vi "parse tcp reply and replace all device var subset.vi"(6 "All device variables array in":string[][](array[string]), 9 "regular expression":string, 10 "String":string, 11 "Clone names and reoplies in":string[][](array[string])) -> (0 "error out":errorcluster, 2 "Device Name":string, 3 "All device variables array":string[][](array[string]), 5 "Clone name and replies array":string[][](array[string]))   [LabVIEW 2020]
panel:
  out "Shot Data parsed array":string[][](array[string])
  out "tcp reply":string
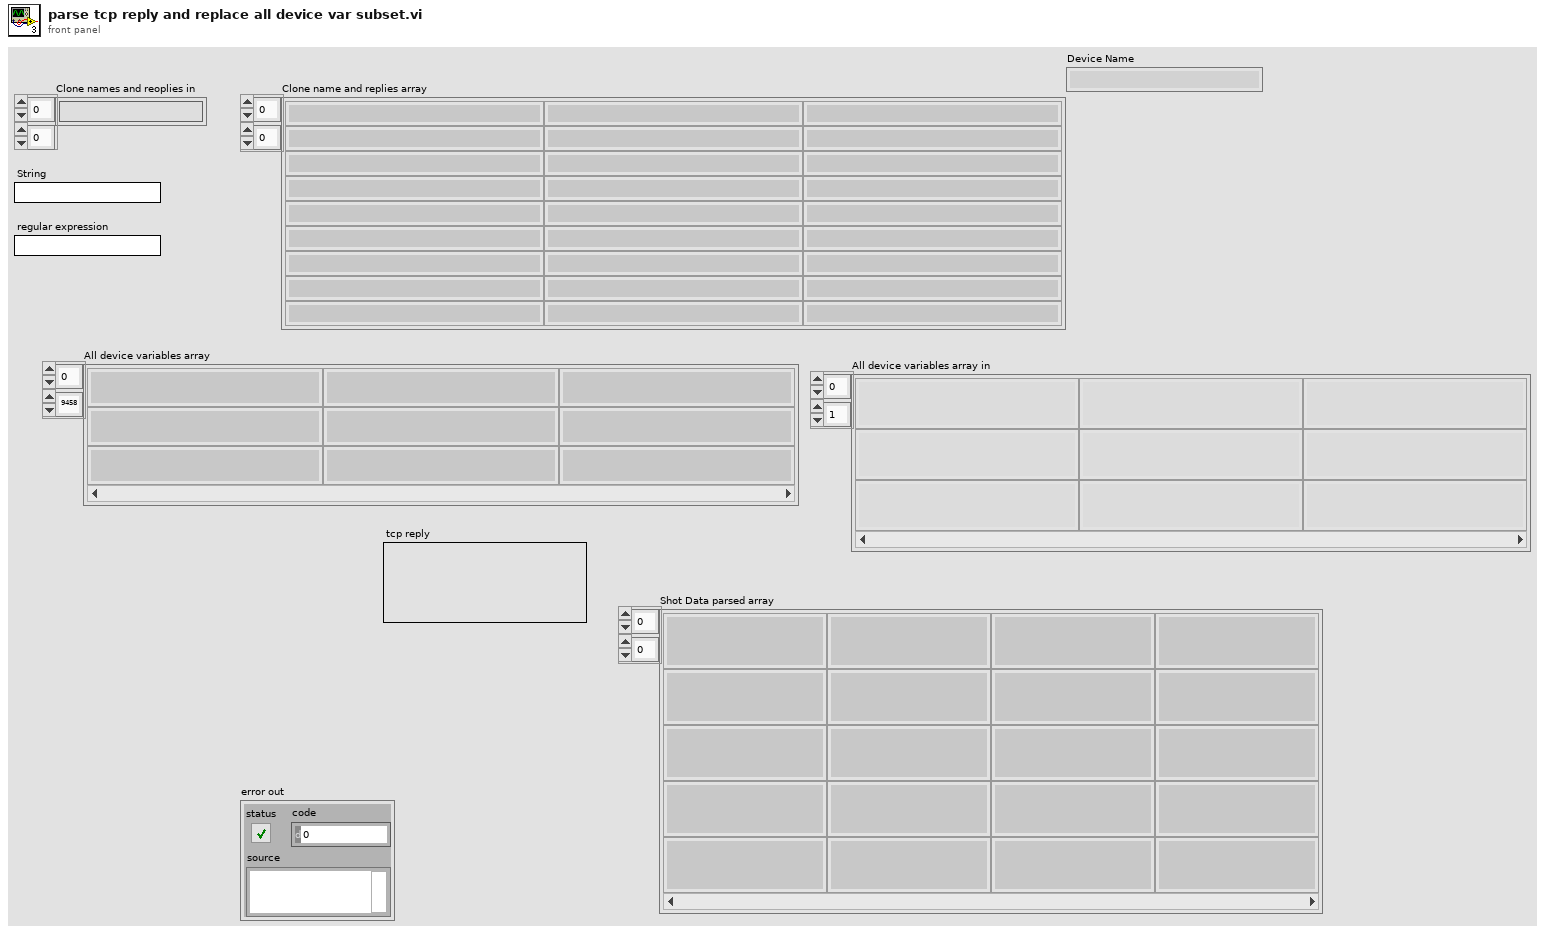
[diagram p1: front panel]
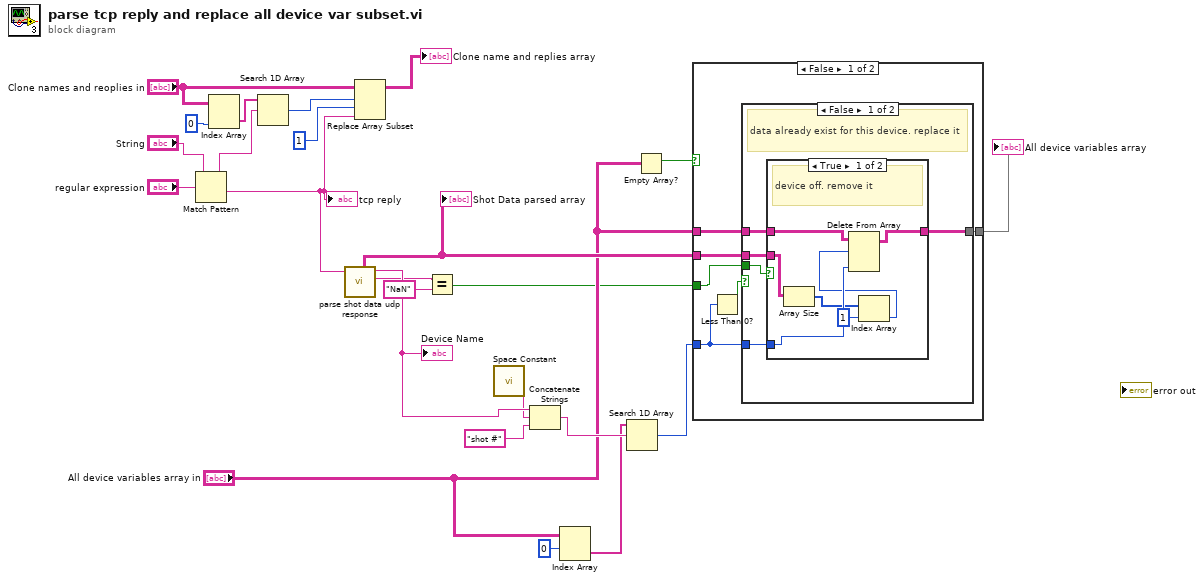
[diagram p0: block diagram]
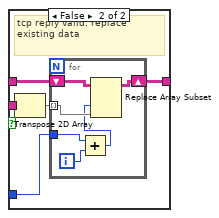
[diagram p2: hidden frame]
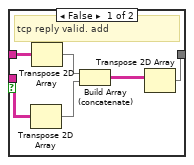
[diagram p4: hidden frame]
diagram:
  n1 = Match Pattern(string="String", regular expression="regular expression") -> (before substring=w24:string, after substring=w16:string)  [unwired: 1 in, 2 out]
  "tcp reply" <- w16
  n2 = Index Array(array="Clone names and reoplies in", index (col)=0 ("disabled index (col)")) -> (element=w19:string[])  [unwired: 1 in]
  n3 = Search 1D Array(1D array=w19, element=w24) -> (index of element=w14:i32)  [unwired: 1 in]
  n4 = call "parse shot data udp response.vi"("ShotData UDP response"=w16) -> ("shot #"=w3:string, "Shot Data parsed array"=w6:string[][], "Device Name"=w8:string)  [unwired: 2 in, 3 out]
  "Shot Data parsed array" <- w6
  "Device Name" <- w8
  n5 = Replace Array Subset(array="Clone names and reoplies in", new element=w16, index (row)=w14, index (col)=1 ("disabled index (col)")) -> (→"Clone name and replies array":string[][])
  n6 = Equal?(x=w3, y="NaN") -> (x = y?=w1:bool)
  n7 = call <vilib>:"Space Constant.vi"() -> ("String"=w7:string)
  n8 = Concatenate Strings(w8, w7, "shot #") -> (w12:string)
  n9 = Index Array(array="All device variables array in", index (row)=0) -> (element=w10:string[])  [unwired: 1 in]
  n10 = Search 1D Array(1D array=w10, element=w12) -> (index of element=w9:i32)  [unwired: 1 in]
  n11 = Empty Array?(array="All device variables array in") -> (empty?=w4:bool)
  n12 = case shown="False" w4 {
    tunnel: [w30 w66] -> w15
    tunnel: w9 -> [w28 _]
    tunnel: w6 -> [w27 w67]
    tunnel: "All device variables array in" -> [w26 w65]
    tunnel: w1 -> [w25 w68]
    frame False {
      n13 = Less Than 0?(x=w28) -> (x < 0?=w29:bool)
      n14 = case shown="False" w29 {
        tunnel: [w35 w56] -> w30
        tunnel: w27 -> [w34 w55]
        tunnel: w26 -> [w33 w57]
        tunnel: w28 -> [w32 _]
        tunnel: w25 -> [w31 w54]
        frame False {
          # "data already exist for this device. replace it"
          n15 = case shown="True" w31 {
            tunnel: [w42 w47] -> w35
            tunnel: w34 -> [w39 w46]
            tunnel: w33 -> [w41 w45]
            tunnel: w32 -> [w40 w44]
            frame True {
              # "device off. remove it"
              n16 = Array Size(array=w39) -> (size(s)=w38:i32[])
              n17 = Index Array(array=w38, index=1) -> (element=w36:i32)
              n18 = Delete From Array(array=w41, length=w36, index (col)=w40) -> (array with subset deleted=w42:string[][])  [unwired: 1 in, 1 out]
            }
            frame False {
              # "tcp reply valid. replace existing data"
              n19 = Transpose 2D Array(2D array=w46) -> (transposed array=w43:string[][])
              n20 = for {
                shift-right: [w52] -> w47
                shift-left: w45 -> [w53]
                tunnel: w43 -> [w51] mode=indexing
                tunnel: w44 -> [w49]
                i -> [w50]
                n21 = Add(x=w49, y=w50) -> (x+y=w48:i32)
                n22 = Replace Array Subset(array=w53, new element=w51, index (col)=w48) -> (w52:string[][])  [unwired: 1 in]
              }
            }
          }
        }
        frame True {
          # "No data exists for this device yet. Append it to the array."
          n23 = case shown="True" w54 {
            tunnel: w57 -> [w63 w64]
            tunnel: [w60 w64] -> w56
            tunnel: w55 -> [w59 _]
            frame False {
              # "tcp reply valid. add"
              n24 = Transpose 2D Array(2D array=w59) -> (transposed array=w58:string[][])
              n25 = Transpose 2D Array(2D array=w63) -> (transposed array=w62:string[][])
              n26 = Build Array (concatenate)(w62, w58) -> (w61:string[][])
              n27 = Transpose 2D Array(2D array=w61) -> (transposed array=w60:string[][])
            }
            frame True {
              # "tcp reply not valid. do nothing"
            }
          }
        }
      }
    }
    frame True {
      # "All dev array empty. pass through the first tcp reply"
      n28 = case shown="False" w68 {
        tunnel: w67 -> [w69 _]
        tunnel: [w69 w70] -> w66
        tunnel: w65 -> [_ w70]
        frame False {
          # "tcp reply valid. pass thru new reply"
        }
        frame True {
          # "tcp timed out (NaN) response\ndo nothing"
        }
      }
    }
  }
  "All device variables array" <- w15
